vi "FlatToRichmicron_MessageReply_Status.vi"(5 "OutputClusterType":T1, 11 "InputCluster":T2) -> (3 "OutputCluster":T1)   [LabVIEW 2019, in "Micron_server.lvlib"]
uses:
  Micron_server.lvlib
  micron_MessageReply_Status_Flat.ctl
  micron_MessageReply_Status.ctl
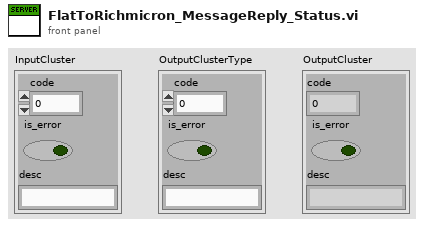
[diagram p1: front panel]
types:
  T1 = typedef "Micron_server.lvlib/micron_MessageReply_Status.ctl" = cluster{"code":i32, "is_error":bool, "desc":string}
  T2 = typedef "Micron_server.lvlib/micron_MessageReply_Status_Flat.ctl" = cluster{"code":i32, "is_error":bool, "desc":string}
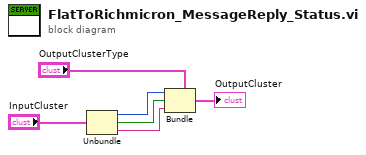
[diagram p0: block diagram]
diagram:
  n1 = Unbundle "Unbundle"("InputCluster") -> ("code"=w3:i32, "is_error"=w2:bool, "desc"=w1:string)
  n2 = Bundle "Bundle"(cluster="OutputClusterType", "code"=w3, "is_error"=w2, "desc"=w1) -> (→"OutputCluster":T1)
